vi "RestoreSetupLVSource.vi"   [LabVIEW 2021]
uses:
  <vilib>/Wiresmith Technology/G CLI/CLI Class/CLI.lvclass
  <userlib>/_OpenG.lib/file/file.llb/openg_file.lvlib
  <vilib>/Utility/config.llb/NI_LVConfig.lvlib
  <userlib>/_OpenG.lib/lvzip/lvzip.llb/subVI/ZLIB Extract All Files To Dir (Path)__ogtk.vi
  <userlib>/_OpenG.lib/file/file.llb/Convert File Extension (Path)__ogtk.vi
  <userlib>/_OpenG.lib/lvzip/fileutil.llb/subVIs/FILE Rename (Path)__ogtk.vi
types:
  T1 = enum32{"Invalid", "Standard", "Closed", "Hidden", "Minimized", "Maximized"}
  T2 = typedef "NI_LVConfig.lvlib/Config Data RefNum.ctl" = refnum<k1>
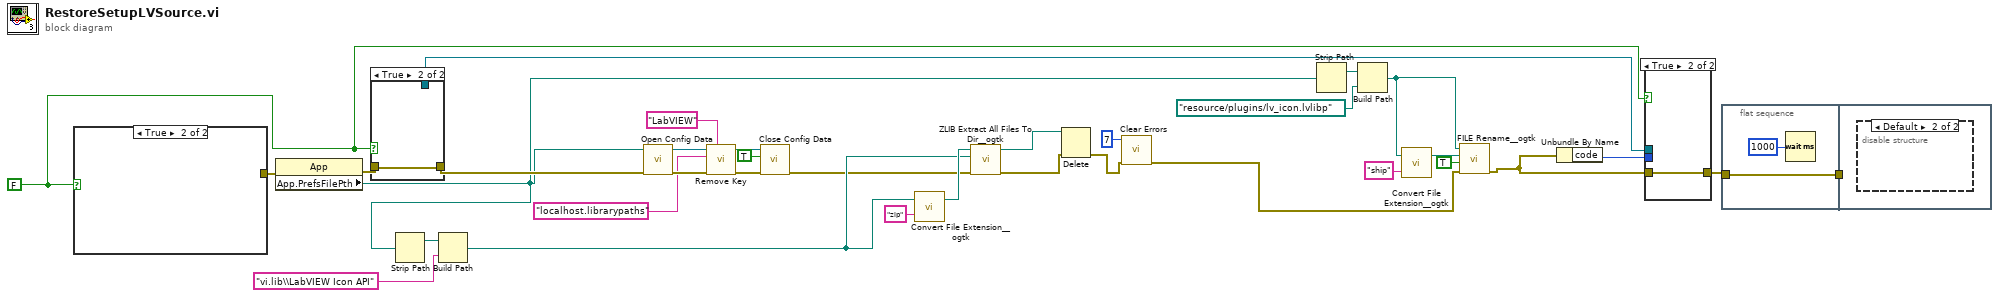
[diagram p0: block diagram]
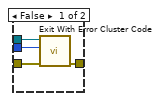
[diagram p2: hidden frame]
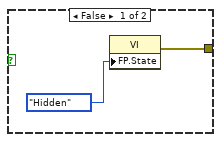
[diagram p3: hidden frame]
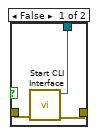
[diagram p4: hidden frame]
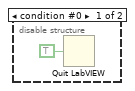
[diagram p5: hidden frame]
diagram:
  w10 = FALSE
  n1 = case shown="True" w10 {
    tunnel: [w35 _] -> w30
    frame False {
      n2 = property class="VI"("FP.State"=T1."Hidden" ("Front Panel Window:State")) -> (error out=w35:errorcluster)  [unwired: 2 in, 1 out]
    }
    frame True {
    }
  }
  n3 = property class="App"(error in=w30) -> (error out=w29:errorcluster, "App.PrefsFilePth"=w1:path)  [unwired: 1 in, 1 out]
  n4 = case shown="True" w10 {
    tunnel: [w39 _] -> w34
    tunnel: w29 -> [w38 w40]
    tunnel: [w37 w40] -> w17
    frame False {
      n5 = call <vilib>:"Start CLI Interface.vi"("error in (no error)"=w38) -> ("error out"=w37:errorcluster, "CLI out"=w39:refnum<class "CLI.lvclass">)  [unwired: 7 in, 2 out]
    }
    frame True {
    }
  }
  n6 = Strip Path(path=w1) -> (stripped path=w26:path)  [unwired: 1 out]
  n7 = Build Path(base path=w26, name or relative path="vi.lib\\LabVIEW Icon API" ("name")) -> (appended path=w24:path)
  n8 = call <vilib>:"Open Config Data.vi"("error in (no error)"=w17, "configuration file path"=w1) -> ("error out"=w21:errorcluster, "refnum"=w19:T2)  [unwired: 7 in, 1 out]
  n9 = call <vilib>:"Remove Key.vi"("section"="LabVIEW", "error in (no error)"=w21, "key"="localhost.librarypaths", "refnum"=w19) -> ("error out"=w20:errorcluster, "refnum out"=w18:T2)  [unwired: 5 in, 1 out]
  n10 = call <vilib>:"Close Config Data.vi"("error in (no error)"=w20, "write file if changed (T)"=TRUE, "refnum"=w18) -> ("error out"=w16:errorcluster)  [unwired: 7 in, 1 out]
  n11 = call-poly <userlib>:"Convert File Extension__ogtk.vi"("new ending (none)"="zip", "file name"=w24) -> ("new filename"=w25:path)  [unwired: 1 out]
  n12 = call-poly <userlib>:"ZLIB Extract All Files To Dir__ogtk.vi"("error in (no error)"=w16, "destination directory (archive name without ending)"=w24, "archive name (file dialog)"=w25) -> ("error out"=w23:errorcluster, "archive name out"=w22:path)  [unwired: 6 in, 1 out]
  n13 = Delete(path (use dialog)=w22, error in=w23) -> (error out=w12:errorcluster)  [unwired: 3 in, 2 out]
  n14 = call <vilib>:"Clear Errors.vi"("error in (no error)"=w12, "specific error code to clear (0: all)"=7) -> ("error out"=w3:errorcluster)  [unwired: 4 in, 1 out]
  n15 = Strip Path(path=w1) -> (stripped path=w9:path)  [unwired: 1 out]
  n16 = Build Path(base path=w9, name or relative path=path "resource/plugins/lv_icon.lvlibp") -> (appended path=w4:path)
  n17 = call-poly <userlib>:"Convert File Extension__ogtk.vi"("new ending (none)"="ship", "file name"=w4) -> ("new filename"=w5:path)  [unwired: 1 out]
  n18 = call-poly <userlib>:"FILE Rename__ogtk.vi"("error in (no error)"=w3, "overwrite (F)"=TRUE, "source path"=w5, "target path"=w4) -> ("error out"=w2:errorcluster)  [unwired: 6 in, 1 out]
  n19 = Unbundle By Name(w2) -> ("code"=w31:i32)
  n20 = case shown="True" w10 {
    tunnel: w34 -> [w44 _]
    tunnel: [w43 w45] -> w32
    tunnel: w31 -> [w42 _]
    tunnel: w2 -> [w41 w45]
    frame False {
      n21 = call <vilib>:"Exit With Error Cluster Code.vi"("error in (no error)"=w41, "No Error Code (0)"=w42, "CLI in"=w44) -> ("error out"=w43:errorcluster)  [unwired: 8 in]
    }
    frame True {
    }
  }
  n22 = flat-sequence {
    tunnel: w32 -> [w47]
    tunnel: [w47] -> w33
    tunnel: w33 -> [_]
    frame #0 {
      n23 = Wait (ms)(milliseconds to wait=u32 1000) -> ()  [unwired: 1 out]
    }
    frame #1 {
      n24 = disable-structure shown="Default" {
        frame condition #0 {
          n25 = Quit LabVIEW(quit? (T)=TRUE) -> ()
        }
        frame condition #1 (active) {
        }
      }
    }
  }
